vi "set_Ga_dilut_cond.vi"(0 "Ga flow (0-10 sccm)":dbl, 1 "fDilution":dbl, 2 "Run":bool, 3 "Bubbler In":bool, 4 "Active":bool) -> ()   [LabVIEW 2011]
panel:
  out "do dilute":bool
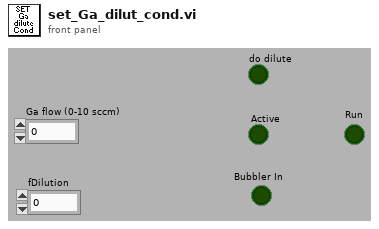
[diagram p1: front panel]
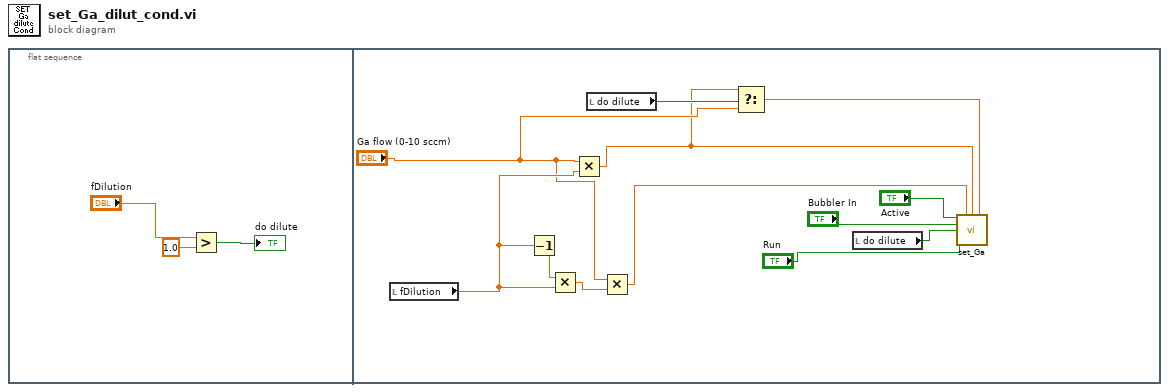
[diagram p0: block diagram]
diagram:
  n1 = flat-sequence {
    frame #0 {
      n2 = Greater?(x="fDilution", y=1.0) -> (0:→"do dilute":bool)
    }
    frame #1 {
      n3 = local read "fDilution"() -> (w15:dbl)
      n4 = Decrement(x=w15) -> (x-1=w10:dbl)
      n5 = Multiply(x=w10, y=w15) -> (x*y=w11:dbl)
      n6 = Multiply(x="Ga flow (0-10 sccm)", y=w15) -> (x*y=w5:dbl)
      n7 = local read "do dilute"() -> (w13:bool)
      n8 = Multiply(x="Ga flow (0-10 sccm)", y=w11) -> (x*y=w4:dbl)
      n9 = Select(t=w5, s=w13, f="Ga flow (0-10 sccm)") -> (s? t:f=w6:dbl)
      n10 = local read "do dilute"() -> (w12:bool)
      n11 = call "set_Ga.vi"("Active"="Active", "GAMFC3"=w4, "GAMFC2"=w5, "GAMFC1"=w6, "Bubbler In"="Bubbler In", "H2 Dilute"=w12, "Run"="Run") -> ()  [unwired: 9 in]
    }
  }
